vi "ZufallFeldGenarator (SubVI).vi"(4 "Numerisch":u8, 5 "BoolArray (Eingang)":bool[][](array[boolean]), 6 "Tic Tac Toe (Eingang)":u8[][](array[numeric]), 7 "Toggle turn (Eingang)":bool) -> (1 "BoolArray (Ausgang)":bool[][](array[boolean]), 2 "Tic Tac Toe (Ausgang)":u8[][](array[numeric]), 3 "Toggle turn (Ausgang)":bool)   [LabVIEW 2017]
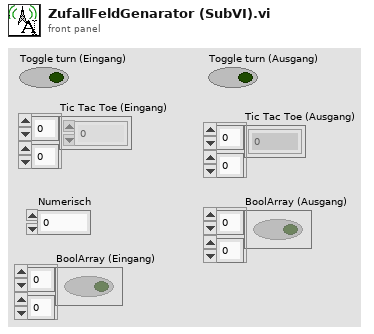
[diagram p1: front panel]
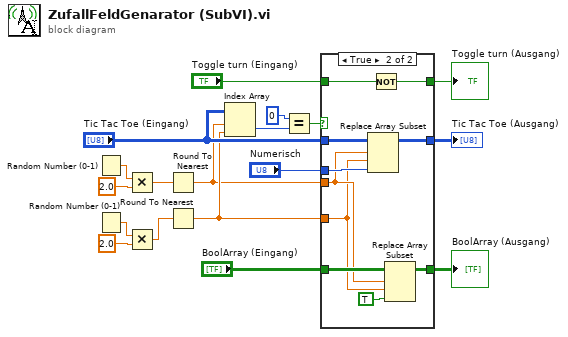
[diagram p0: block diagram]
diagram:
  n1 = Random Number (0-1)() -> (number: 0 to 1=w3:dbl)
  n2 = Random Number (0-1)() -> (number: 0 to 1=w6:dbl)
  n3 = Multiply(x=w3, y=2.0) -> (x*y=w4:dbl)
  n4 = Multiply(x=w6, y=2.0) -> (x*y=w7:dbl)
  n5 = Round To Nearest(number=w4) -> (nearest integer value=w11:dbl)
  n6 = Round To Nearest(number=w7) -> (nearest integer value=w12:dbl)
  n7 = Index Array(array="Tic Tac Toe (Eingang)", index (row)=w11, index (col)=w12) -> (element=w8:u8)
  n8 = Equal?(x=0, y=w8) -> (x = y?=w9:bool)
  n9 = case shown="True" w9 {
    tunnel: [w19 w31] -> w10
    tunnel: "Tic Tac Toe (Eingang)" -> [w21 w30]
    tunnel: w11 -> [_ w25]
    tunnel: w12 -> [_ w24]
    tunnel: "Numerisch" -> [_ w29]
    tunnel: [w21 w28] -> w17
    tunnel: "BoolArray (Eingang)" -> [w20 w26]
    tunnel: [w20 w27] -> w13
    tunnel: "Toggle turn (Eingang)" -> [w19 w23]
    frame False {
    }
    frame True {
      n10 = Replace Array Subset(array=w30, new element=w29, index (row)=w25, index (col)=w24) -> (w28:u8[][])
      n11 = Not(x=w23) -> (.not. x?=w31:bool)
      n12 = Replace Array Subset(array=w26, new element=TRUE ("Neues Element/Teil-Array"), index (row)=w25, index (col)=w24) -> (w27:bool[][])
    }
  }
  "Tic Tac Toe (Ausgang)" <- w17
  "BoolArray (Ausgang)" <- w13
  "Toggle turn (Ausgang)" <- w10
